vi "GetLocalCameras.vi"(8 "error in (no error)":errorcluster) -> (0 "error out":errorcluster, 3 "Camera Information Array":T1(array[cluster]))   [LabVIEW 2017, in "IrManageCameras.lvlib"]
uses:
  <vilib>/addons/InsightCM/Devices/Shared/Ir/IrManageCameras/IrManageCameras.lvlib
  <vilib>/vision/driver/NI_Vision_Acquisition_Software.lvlib
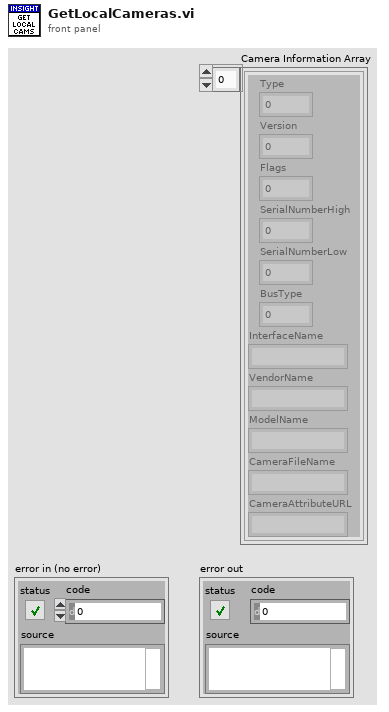
[diagram p1: front panel]
types:
  T1 = cluster{"Type":u32, "Version":u32, "Flags":u32, "SerialNumberHigh":u32, "SerialNumberLow":u32, "BusType":u32, "InterfaceName":string, "VendorName":string, "ModelName":string, "CameraFileName":string, "CameraAttributeURL":string}[]
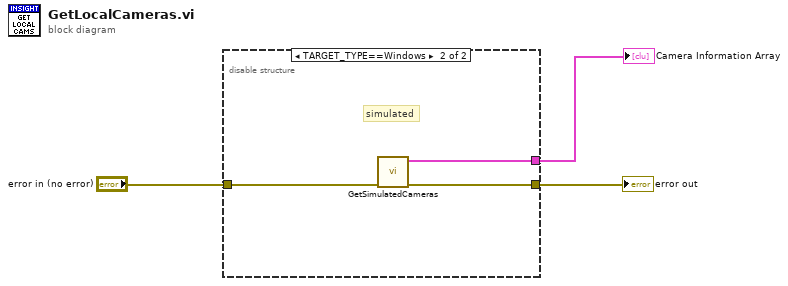
[diagram p0: block diagram]
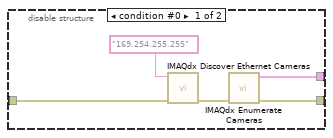
[diagram p2: hidden frame]
diagram:
  n1 = disable-structure shown="TARGET_TYPE==Windows" {
    disable-tunnel: [w6 w11] -> w1
    disable-tunnel: [w5 w9] -> w2
    disable-tunnel: "error in (no error)" -> [w4 w10]
    frame condition #0 {
      n2 = call <vilib>:"IMAQdx Discover Ethernet Cameras.vi"("error in"=w4, "Address (Broadcast)"="169.254.255.255") -> ("error out"=w8:errorcluster)  [unwired: 9 in]
      n3 = call <vilib>:"IMAQdx Enumerate Cameras.vi"("error in"=w8) -> ("error out"=w6:errorcluster, "Camera Information Array"=w5:T1)  [unwired: 9 in]
    }
    frame condition #1 (active) {
      # "simulated"
      n4 = call <vilib>:"GetSimulatedCameras.vi"("error in (no error)"=w10) -> ("error out"=w11:errorcluster, "Camera Info"=w9:T1)  [unwired: 9 in]
    }
  }
  "Camera Information Array" <- w2
  "error out" <- w1
